vi "Demo4-Set_Values.vi"() -> ()   [LabVIEW 2020]
panel:
  in  "Set All":bool
  in  "Set Values\n(Fully empty cells will not be set)":string[](array[string])
  out "Live Readback Values":string[](array[string])
  out "Settable Device Keywords":string[](array[string])
  in  "IP Address of Remote Device":string="196.254.31.200"
  in  "Disconnect":bool
  # "Diode Demo - Set Values"
  # "Demonstrates setting parameters for the STM32 Diode Device."
  # "VI Instructions\n\n1. Make sure you know the Device IP Address.\n2. From Windows command prompt, confirm ping to IP address.\n3. Type the correct device IP address into this VI.\n3. Run this VI. *Note:* Only one TCP connection to the device's SCPI-like server can run at a time.\n4. When finished, disconnect safely from the device via the \"Disconnect\" toggle button. (Not the Abort button).\n\nCreated by Scott Feister on July 13, 2022."
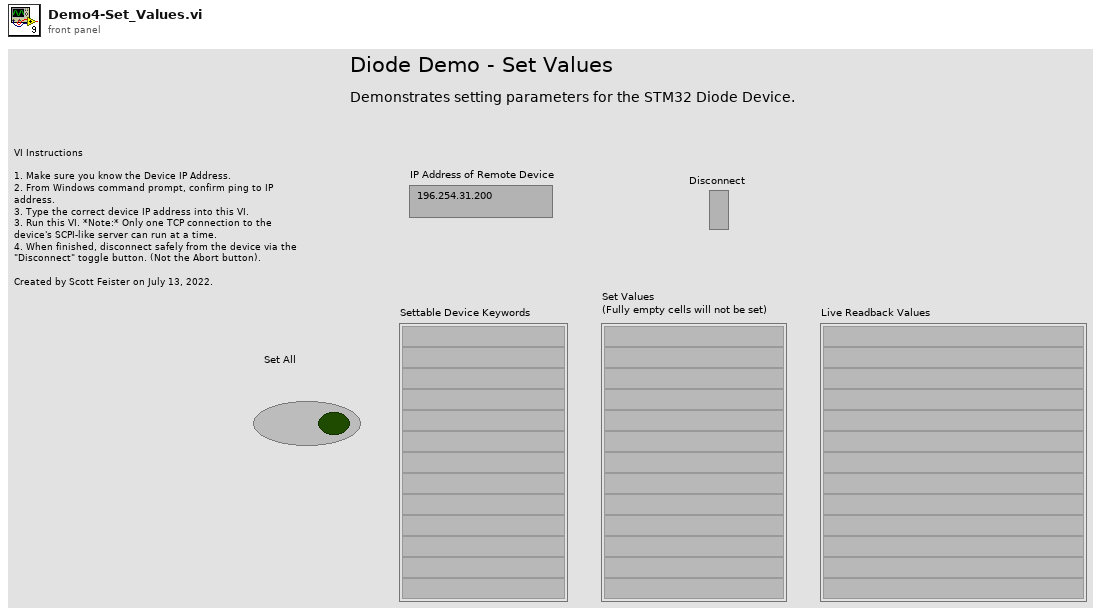
[diagram p1: front panel]
types:
  T1 = typedef "DDAQ-Keyword.ctl" = cluster{"Keyword":string, "Gettable":bool, "Settable":bool, "Is Array":bool, "Data Type":string, "Description":string}
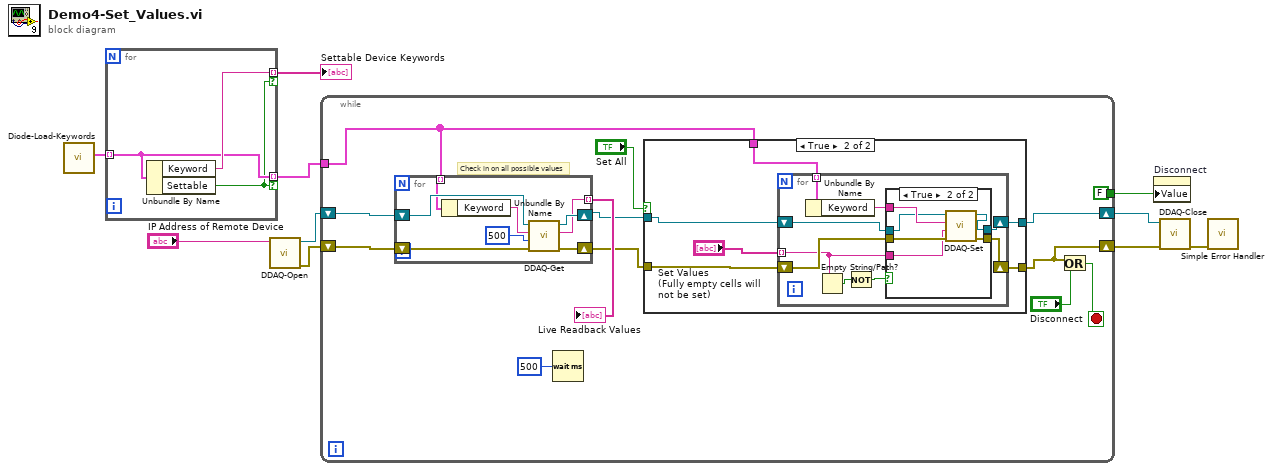
[diagram p0: block diagram]
diagram:
  n1 = call "Diode-Load-Keywords.vi"() -> ("Diodes Keywords Array"=w3:T1[])  [unwired: 11 in]
  n2 = for {
    tunnel: w3 -> [w12] mode=indexing
    tunnel: [w13] -> w2 mode=indexing if=w11
    tunnel: [w12] -> w1 mode=indexing if=w11
    n3 = Unbundle By Name(w12) -> ("Keyword"=w13:string, "Settable"=w11:bool)
  }
  "Settable Device Keywords" <- w2
  n4 = call "DDAQ-Open.vi"("IP Address of Nucleo Device"="IP Address of Remote Device") -> ("error out"=w9:errorcluster, "connection ID"=w10:refnum<k5>)  [unwired: 9 in]
  n5 = while {
    shift-right: [w14] -> w8
    shift-left: w10 -> [w26]
    shift-right: [w15] -> w7
    shift-left: w9 -> [w25]
    tunnel: [FALSE] -> w5
    tunnel: w1 -> [w18]
    stop <- w21 stop-if-true
    # "Check in on all possible values"
    n6 = for {
      shift-right: [w57] -> w17
      shift-left: w26 -> [w59]
      shift-right: [w56] -> w16
      shift-left: w25 -> [w58]
      tunnel: [w54] -> w20 mode=indexing
      tunnel: w18 -> [w53] mode=indexing
      n7 = Unbundle By Name(w53) -> ("Keyword"=w52:string)
      n8 = call "DDAQ-Get.vi"("error in (no error)"=w58, "max bytes to read (10000)"=500 ("max bytes to read (500)"), "SCPI-like Keyword (leave off question mark)"=w52, "connection ID"=w59) -> ("error out"=w56:errorcluster, "Response"=w54:string, "connection ID out"=w57:refnum<k5>)  [unwired: 4 in, 1 out]
    }
    "Live Readback Values" <- w20
    n9 = Wait (ms)(milliseconds to wait=u32 500) -> ()  [unwired: 1 out]
    n10 = case shown="True" "Set All" {
      tunnel: w18 -> [_ w33]
      tunnel: w17 -> [w27 w32]
      tunnel: w16 -> [w28 w31]
      tunnel: [w28 w30] -> w15
      tunnel: [w27 w29] -> w14
      frame False {
      }
      frame True {
        n11 = for {
          tunnel: "Set Values\n(Fully empty cells will not be set)" -> [w35] mode=indexing
          tunnel: w33 -> [w43] mode=indexing
          shift-right: [w37] -> w30
          shift-left: w31 -> [w38]
          shift-right: [w36] -> w29
          shift-left: w32 -> [w41]
          n12 = Unbundle By Name(w43) -> ("Keyword"=w42:string)
          n13 = Empty String/Path?(string/path=w35) -> (empty?=w39:bool)
          n14 = Not(x=w39) -> (.not. x?=w40:bool)
          n15 = case shown="True" w40 {
            tunnel: w42 -> [_ w51]
            tunnel: w41 -> [w44 w50]
            tunnel: w38 -> [w45 w49]
            tunnel: [w45 w48] -> w37
            tunnel: [w44 w47] -> w36
            tunnel: w35 -> [_ w46]
            frame False {
            }
            frame True {
              n16 = call "DDAQ-Set.vi"("error in (no error)"=w49, "Set Value"=w46, "SCPI-like Keyword (leave off space, value)"=w51, "connection ID"=w50) -> ("error out"=w48:errorcluster, "connection ID out"=w47:refnum<k5>)  [unwired: 6 in]
            }
          }
        }
      }
    }
    n17 = Or(x=w15, y="Disconnect") -> (x .or. y?=w21:bool)
  }
  n18 = property on="Disconnect" class="Bool (strict)"("Value"=w5) -> ()  [unwired: 2 in, 2 out]
  n19 = call "DDAQ-Close.vi"("error in (no error)"=w7, "connection ID"=w8) -> ("error out"=w6:errorcluster)  [unwired: 9 in]
  n20 = call <vilib>:"Simple Error Handler.vi"("error in (no error)"=w6) -> ()  [unwired: 4 in, 5 out]
